vi "TimerWithDAQmx.vi"(9 "Condition (>condition Fire and TTL)":dbl=10.0, 10 "Period (Sec)":dbl=20.0 format="%#_13g", 11 "milliseconds to wait":u32=1000) -> ()   [LabVIEW 2018]
uses:
  <vilib>/DAQmx/write.llb/DAQmx Write (Digital Bool 1Line 1Point).vi
  <vilib>/DAQmx/create/channels.llb/DAQmx Create Channel (DO-Digital Output).vi
  <vilib>/DAQmx/miscellaneous.llb/DAQmx Fill In Error Info.vi
panel:
  out "error out":errorcluster
  out "PulseNumber Now":dbl=14.0
  out "Pulse Number":dbl=5.0
  out "Waveform Chart":i32(graph)
  out "floor(x/y) 2":i32=1
  out "floor(x/y)":dbl=2.0
  out "TTL ?":bool
  out "Time Index":i32=2
  in  "stop 3":bool
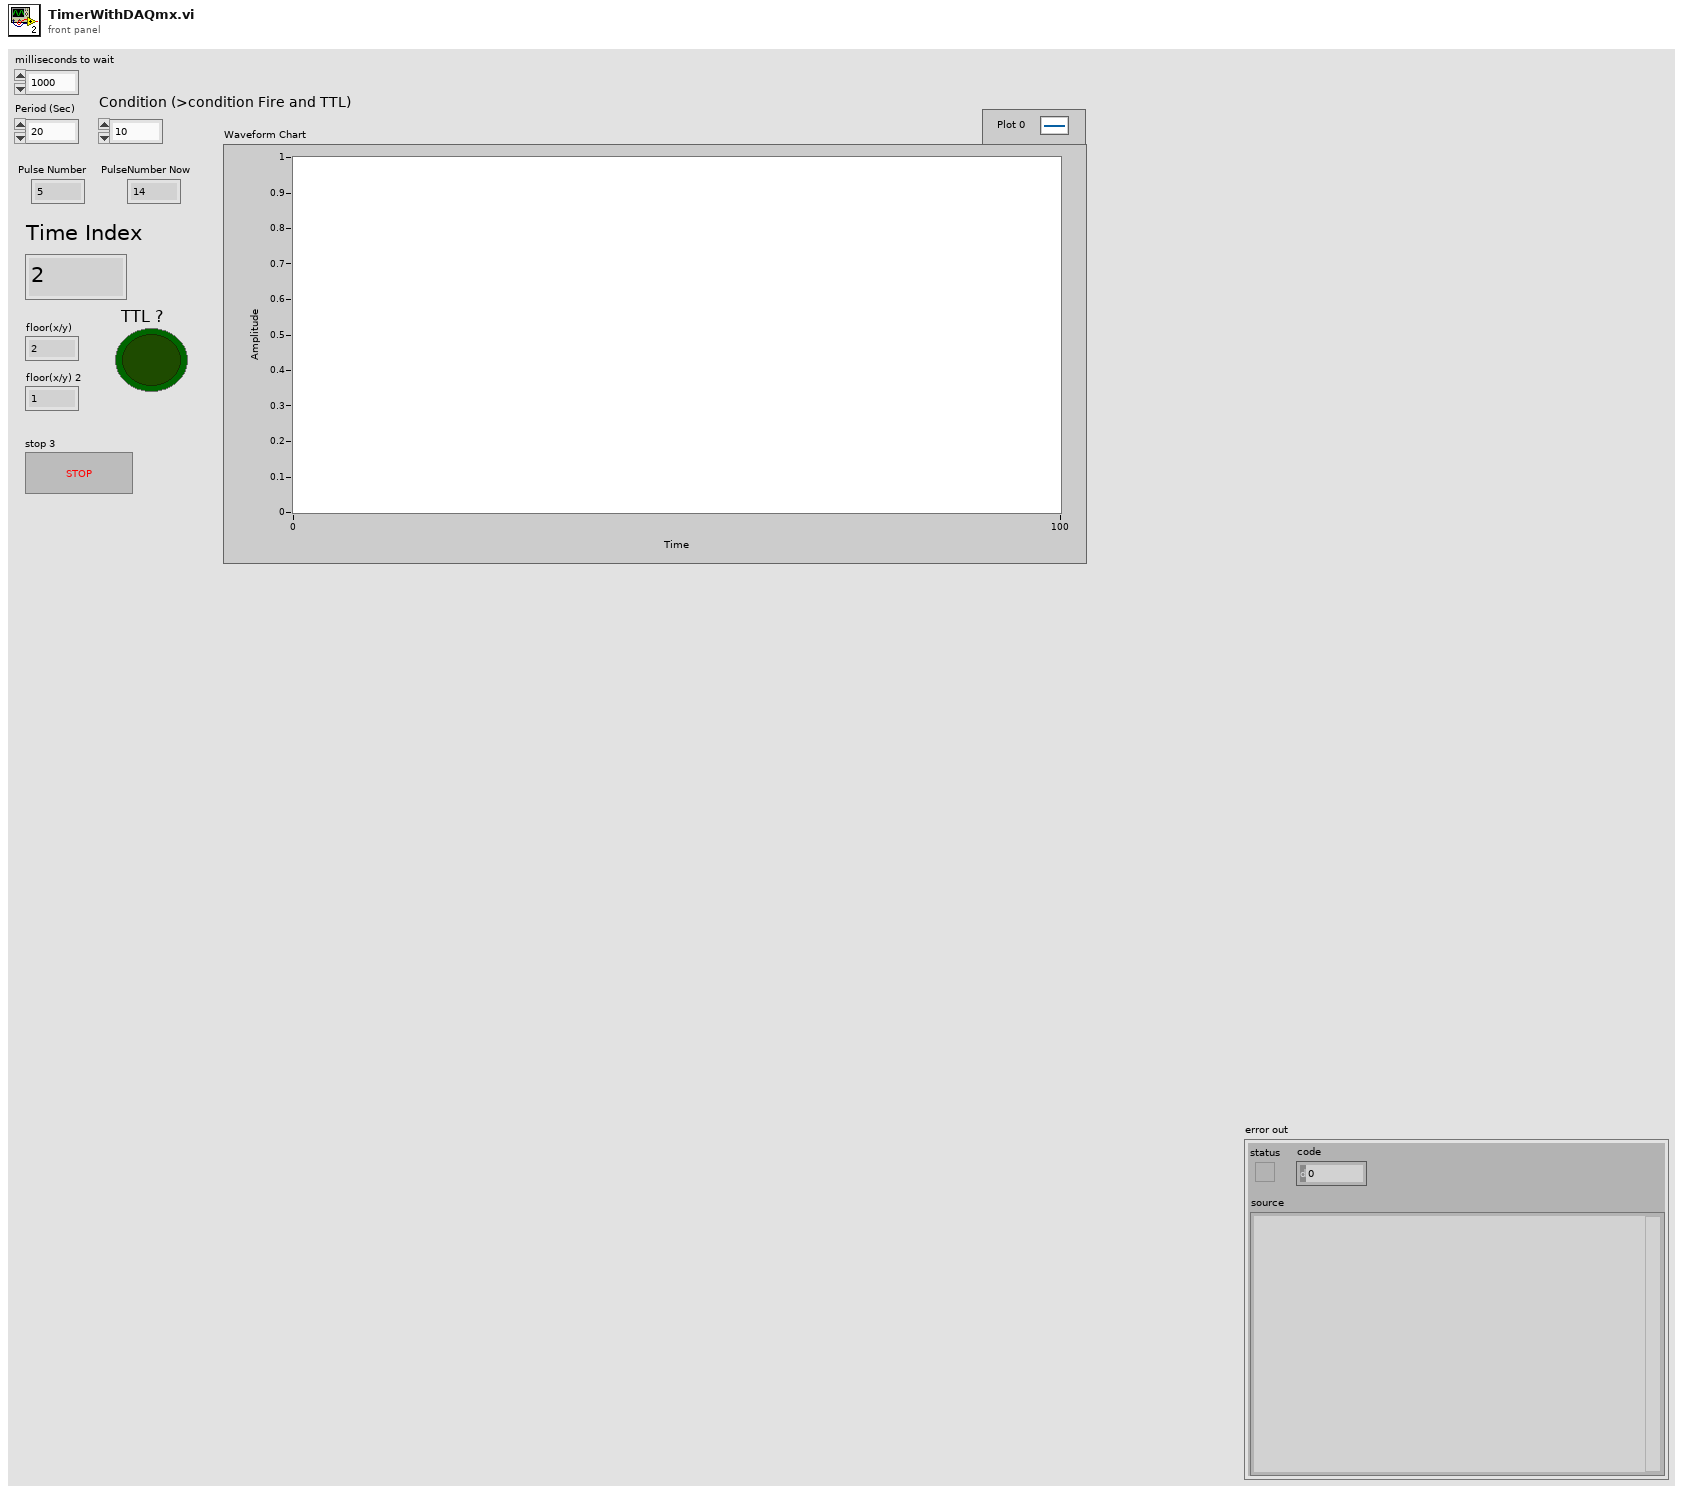
[diagram p1: front panel]
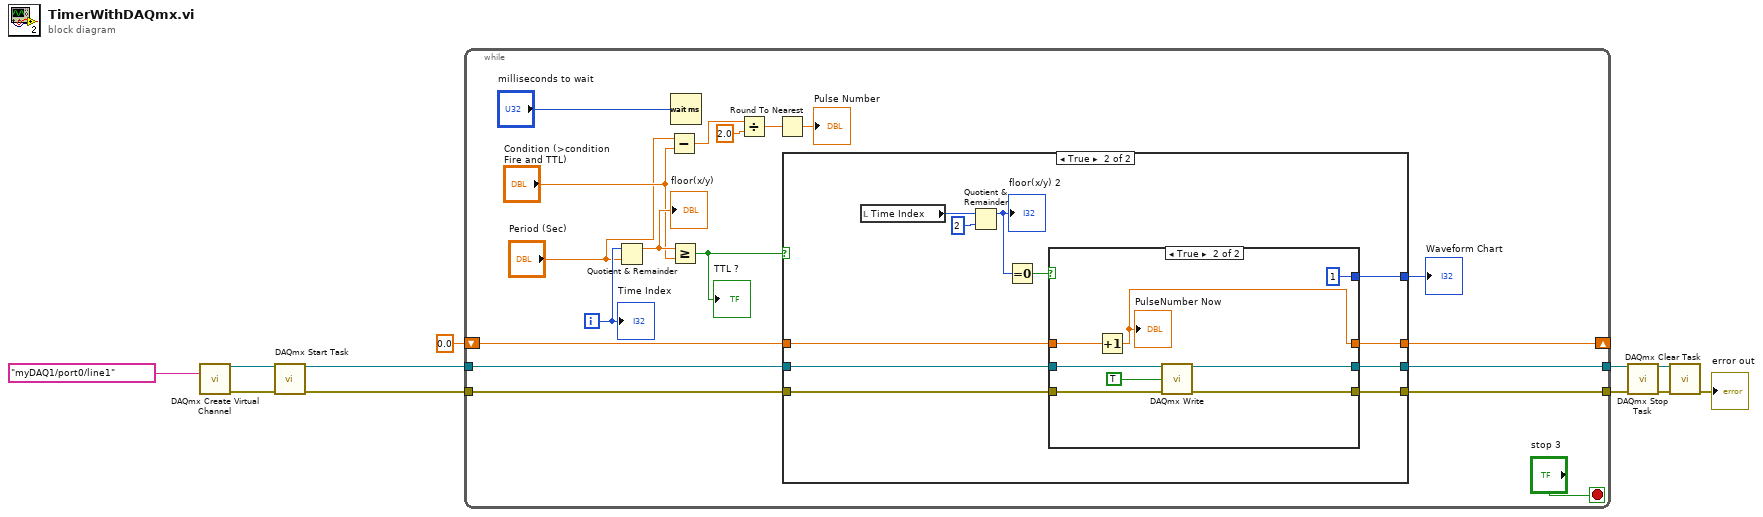
[diagram p0: block diagram]
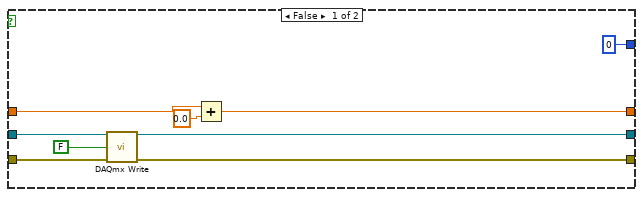
[diagram p2: hidden frame]
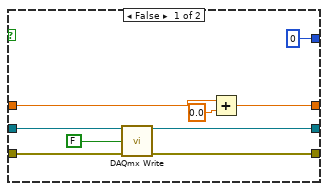
[diagram p3: hidden frame]
diagram:
  n1 = call-poly <vilib>:"DAQmx Create Virtual Channel.vi"("lines"=tag "myDAQ1/port0/line1") -> ("task out"=w10:refnum<k21>, "error out"=w9:errorcluster)  [unwired: 13 in]
  n2 = call <vilib>:"DAQmx Start Task.vi"("task/channels in"=w10, "error in"=w9) -> ("task out"=w7:refnum<k21>, "error out"=w6:errorcluster)  [unwired: 12 in]
  n3 = while {
    shift-right: [w17] -> _
    shift-left: 0.0 -> [w16]
    tunnel: w7 -> [w15]
    tunnel: w6 -> [w14]
    tunnel: [w13] -> w2
    tunnel: [w12] -> w1
    i -> [w27]
    stop <- "stop 3" stop-if-true
    n4 = Quotient & Remainder(x=w27, y="Period (Sec)") -> (x-y*floor(x/y)=w26:dbl)  [unwired: 1 out]
    "floor(x/y)" <- w26
    n5 = Subtract(x="Period (Sec)", y="Condition (>condition Fire and TTL)") -> (x-y=w22:dbl)
    n6 = Greater Or Equal?(x=w26, y="Condition (>condition Fire and TTL)") -> (x >= y?=w25:bool)
    "TTL ?" <- w25
    n7 = Wait (ms)(milliseconds to wait="milliseconds to wait") -> ()  [unwired: 1 out]
    n8 = Divide(x=w22, y=2.0) -> (x/y=w20:dbl)
    n9 = Round To Nearest(number=w20) -> (nearest integer value=→"Pulse Number":dbl)
    n10 = case shown="True" w25 {
      tunnel: [0 w45] -> w24
      tunnel: [w35 w44] -> w17
      tunnel: w16 -> [w36 w43]
      tunnel: w15 -> [w31 w42]
      tunnel: w14 -> [w34 w41]
      tunnel: [w32 w40] -> w13
      tunnel: [w33 w39] -> w12
      frame False {
        n11 = call-poly <vilib>:"DAQmx Write.vi"("task/channels in"=w31, "data"=FALSE, "error in"=w34) -> ("task out"=w32:refnum<k21>, "error out"=w33:errorcluster)  [unwired: 10 in, 1 out]
        n12 = Add(x=w36, y=0.0) -> (x+y=w35:dbl)
      }
      frame True {
        n13 = local read "Time Index"() -> (w49:i32)
        n14 = Quotient & Remainder(x=w49, y=2) -> (x-y*floor(x/y)=w46:i32)  [unwired: 1 out]
        "floor(x/y) 2" <- w46
        n15 = Equal To 0?(x=w46) -> (x = 0?=w48:bool)
        n16 = case shown="True" w48 {
          tunnel: [0 1] -> w45
          tunnel: [w55 w65] -> w44
          tunnel: w43 -> [w57 w64]
          tunnel: w42 -> [w51 w63]
          tunnel: w41 -> [w54 w62]
          tunnel: [w52 w61] -> w40
          tunnel: [w53 w60] -> w39
          frame False {
            n17 = call-poly <vilib>:"DAQmx Write.vi"("task/channels in"=w51, "data"=FALSE, "error in"=w54) -> ("task out"=w52:refnum<k21>, "error out"=w53:errorcluster)  [unwired: 10 in, 1 out]
            n18 = Add(x=w57, y=0.0) -> (x+y=w55:dbl)
          }
          frame True {
            n19 = Increment(x=w64) -> (x+1=w65:dbl)
            "PulseNumber Now" <- w65
            n20 = call-poly <vilib>:"DAQmx Write.vi"("task/channels in"=w63, "data"=TRUE, "error in"=w62) -> ("task out"=w61:refnum<k21>, "error out"=w60:errorcluster)  [unwired: 10 in, 1 out]
          }
        }
      }
    }
    "Waveform Chart" <- w24
    "Time Index" <- w27
  }
  n21 = call <vilib>:"DAQmx Stop Task.vi"("task/channels in"=w2, "error in"=w1) -> ("task out"=w5:refnum<k21>, "error out"=w4:errorcluster)  [unwired: 12 in]
  n22 = call <vilib>:"DAQmx Clear Task.vi"("task in"=w5, "error in"=w4) -> ("error out"=→"error out":errorcluster)  [unwired: 13 in]
